vi "Emergency Query.vi"() -> (3 "Enum":T1)   [LabVIEW 2020]
uses:
  Estados.ctl
  Variables Globales.vi
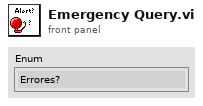
[diagram p1: front panel]
types:
  T1 = typedef "Estados.ctl" = enum16{"Errores?", "Control de válvula", "Nivel bajo?", "Query nivel del tanque", "Query peso del pote", "Ajuste?", "Llenado?", "Emergencia?", "Init", "Ajuste", "Nivel Bajo", "Llenado", "Error", "Emergencia"}
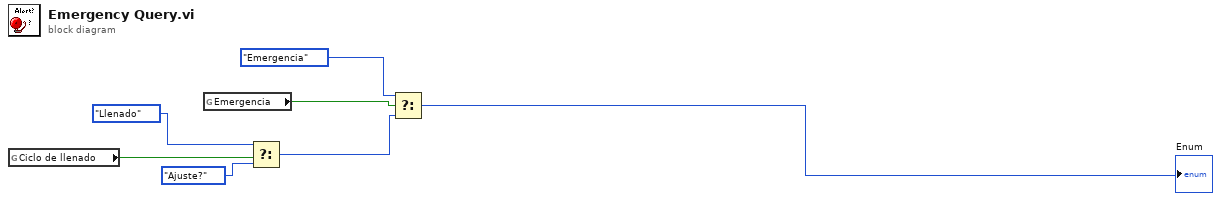
[diagram p0: block diagram]
diagram:
  n1 = global read "Variables Globales.vi" "Ciclo de llenado"() -> (w7:bool)
  n2 = global read "Variables Globales.vi" "Emergencia"() -> (w1:bool)
  n3 = Select(t=Estados."Llenado", s=w7, f=Estados."Ajuste?") -> (s? t:f=w5:T1)
  n4 = Select(t=Estados."Emergencia", s=w1, f=w5) -> (s? t:f=→"Enum":T1)
